vi "picoharp_corr_test.vi"() -> ()   [LabVIEW 2015, in "picoharp.lvclass"]
uses:
  picoharp.lvclass
  Hydraharp/hydraharp/hydraharp_correlation_lag_settings.ctl
  Hydraharp/hydraharp/hydraharp_time_decades.ctl
  Hydraharp/hydraharp_panel/hpanel_acq_modes.ctl
  Hydraharp/hydraharp/hydraharp_action_on_records.ctl
  picoharp.lvclass/picoharp.ctl
panel:
  out "elements_in_record_buffers":i32[](array[numeric])
  out "XY Graph":T1(graph)
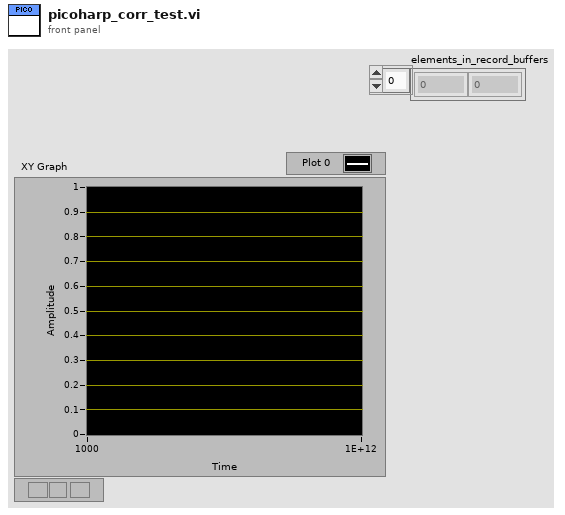
[diagram p1: front panel]
types:
  T1 = cluster{"lags":dbl[], "computed_correlation":dbl[]}[]
  T2 = typedef "hydraharp_action_on_records.ctl" = enum16{"stream_to_file", "correlate", "stream to file and correlate"}
  T3 = typedef "hpanel_acq_modes.ctl" = u16
  T4 = typedef "hydraharp_correlation_lag_settings.ctl" = cluster{"time_start":T5, "time_end":T5, "coarseness":i64}
  T5 = typedef "hydraharp_time_decades.ctl" = i64
  T6 = enum16{"big-endian, network order", "native, host order", "little-endian"}
  T7 = cluster{"log_bin_edges":dbl[], "normalized_correlation":dbl[]}
  T8 = cluster{"log_bin_edges":dbl[], "normalized_correlation":dbl[]}[]
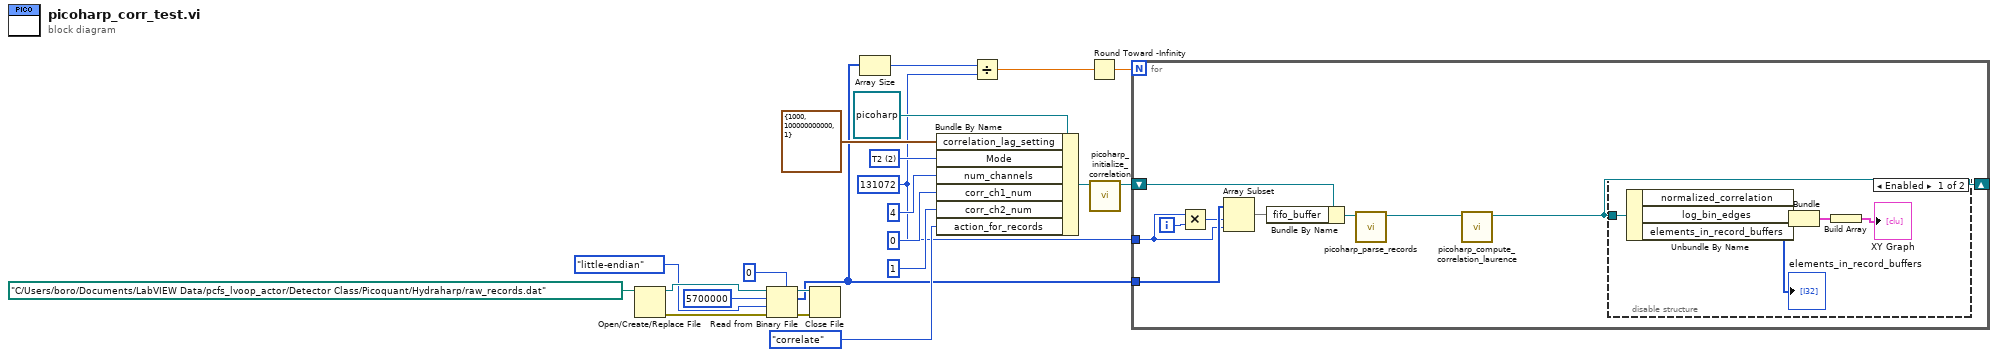
[diagram p0: block diagram]
diagram:
  w2 = 131072 ("y")
  w12 = T3 2 items=["T2"=2, "T3"=3] ("Mode")
  n1 = Open/Create/Replace File(file path (use dialog)=path "C:/Users/boro/Documents/LabVIEW Data/pcfs_lvoop_actor/Detector Class/Picoquant/Hydraharp/raw_records.dat") -> (refnum out=w21:refnum<file>, error out=w17:errorcluster)  [unwired: 5 in, 1 out]
  n2 = Read from Binary File(5:u32 0, 8:w17, 9:T6."little-endian" ("byte order (0:big-endian, network order)"), 10:5700000 ("count (1)"), 11:w21) -> (0:w16:errorcluster, 2:w5:u32[], 3:w18:refnum<file>)  [unwired: 1 in, 1 out]
  n3 = Close File(refnum=w18, error in=w16) -> ()  [unwired: 2 out]
  n4 = Array Size(array=w5) -> (size(s)=w4:i32)
  n5 = Bundle By Name(cluster=refnum<class "picoharp.lvclass"> refnum ("hydraharp in"), "correlation_lag_setting"=T4 {"time_start"=1000, "time_end"=100000000000, "coarseness"=1}, "Mode"=w12, "num_channels"=4, "corr_ch1_num"=0, "corr_ch2_num"=1, "action_for_records"=hydraharp_action_on_records."correlate") -> (w7:refnum<class "picoharp.lvclass">)
  n6 = Divide(x=w4, y=w2) -> (x/y=w3:dbl)
  n7 = Round Toward -Infinity(1:w3) -> (0:w1:dbl)
  n8 = call "picoharp_initialize_correlation.vi"("hydraharp in"=w7) -> ("hydraharp out"=w6:refnum<class "picoharp.lvclass">)  [unwired: 9 in, 1 out]
  n9 = for {
    N: w1 -> [_]
    shift-right: [w23] -> _
    shift-left: w6 -> [w31]
    tunnel: w5 -> [w29]
    tunnel: w2 -> [w25]
    i -> [w27]
    n10 = Multiply(x=w25, y=w27) -> (x*y=w26:i32)
    n11 = Array Subset(array=w29, index=w26, length=w25) -> (w28:u32[])
    n12 = Bundle By Name(cluster=w31, "fifo_buffer"=w28) -> (w30:refnum<class "picoharp.lvclass">)
    n13 = call "picoharp_parse_records.vi"("hydraharp in"=w30) -> ("hydraharp out"=w24:refnum<class "picoharp.lvclass">)  [unwired: 9 in, 1 out]
    n14 = call "picoharp_compute_correlation_laurence.vi"("hydraharp in"=w24) -> ("hydraharp out"=w23:refnum<class "picoharp.lvclass">)  [unwired: 9 in, 1 out]
    n15 = disable-structure shown="Enabled" {
      disable-tunnel: w23 -> [w33 _]
      frame Enabled {
        n16 = Unbundle By Name(w33) -> ("normalized_correlation"=w36:dbl[], "log_bin_edges"=w37:dbl[], "elements_in_record_buffers"=→"elements_in_record_buffers":i32[])
        n17 = Bundle("log_bin_edges"=w37, "normalized_correlation"=w36) -> (w35:T7)  [unwired: 1 in]
        n18 = Build Array(w35) -> (→"XY Graph":T8)
      }
      frame Disabled {
      }
    }
  }
